vi "Register.vi"(8 "error in (no error)":errorcluster, 11 "Test Executive Builder Model in":refnum<class "Test Executive Builder Model.lvclass">) -> (0 "error out":errorcluster, 3 "Test Executive Builder Model out":refnum<class "Test Executive Builder Model.lvclass">)   [LabVIEW 2017, in "Test Executive Builder Model.lvclass"]
uses:
  Test Executive Builder Model.lvclass
  Test Executive Builder Model Messages/Load Test Executive Msg/Load Test Executive Msg.lvclass
  <vilib>/gpm_packages/@cs/mva-core/Source/IObserver/IObserver/IObserver.lvclass
  <vilib>/gpm_packages/@cs/mva-core/Source/SubscriptionPolicy/BasicSubscription/BasicSubscription.lvclass
  Test Executive Builder Model Messages/Insert While Loop Msg/Insert While Loop Msg.lvclass
  Application Dependencies/Insert While Loop.ctl
  Test Executive Builder Model Messages/Insert For Loop Msg/Insert For Loop Msg.lvclass
  Application Dependencies/Insert For Loop.ctl
  Test Executive Builder Model Messages/Insert Stop Loop Msg/Insert Stop Loop Msg.lvclass
  Application Dependencies/Insert Stop Loop.ctl
  Test Executive Builder Model Messages/Insert Test Step Msg/Insert Test Step Msg.lvclass
  Application Dependencies/Insert Test Step.ctl
  Test Executive Builder Model Messages/Insert Subroutine Msg/Insert Subroutine Msg.lvclass
  Application Dependencies/Insert Subroutine.ctl
  Test Executive Builder Model Messages/Insert Subsequence Msg/Insert Subsequence Msg.lvclass
  Application Dependencies/Insert Subsequence.ctl
  Test Executive Builder Model Messages/Insert Conditional Msg/Insert Conditional Msg.lvclass
  Application Dependencies/Insert Conditional.ctl
  Test Executive Builder Model Messages/Remove Element Msg/Remove Element Msg.lvclass
  Test Executive Builder Model Messages/Move or Copy Element Msg/Move or Copy Element Msg.lvclass
  Application Dependencies/Move or Copy Element.ctl
  Test Executive Builder Model Messages/Save Test Executive Msg/Save Test Executive Msg.lvclass
  Test Executive Builder Model Messages/Clear Test Executive Msg/Clear Test Executive Msg.lvclass
  Test Executive Builder Model Messages/Create Test Executive Msg/Create Test Executive Msg.lvclass
  Application Dependencies/Create Test Executive.ctl
  Test Executive Builder Model Messages/Handle Double Click on Element Msg/Handle Double Click on Element Msg.lvclass
  Test Executive Builder Model Messages/Drop Element Msg/Drop Element Msg.lvclass
  Application Dependencies/Drop Element.ctl
  Application Dependencies/Insert Case Structure.ctl
  Test Executive Builder Model Messages/Insert Case Structure Msg/Insert Case Structure Msg.lvclass
  Application Dependencies/Insert Halt.ctl
  Test Executive Builder Model Messages/Insert Halt Msg/Insert Halt Msg.lvclass
  Test Executive Builder Model Messages/Mass Relink Msg/Mass Relink Msg.lvclass
  Test Executive Builder Model Messages/Insert Parallel Msg/Insert Parallel Msg.lvclass
  C:/Program Files/National Instruments/LabVIEW 2017/vi.lib/gpm_packages/@cs/mva-core/Source/IModel/IModel/IModel.lvclass
  C:/Program Files/National Instruments/LabVIEW 2017/vi.lib/gpm_packages/@cs/mva-core/Source/IObserver/IObserver/IObserver.lvclass
  C:/Program Files/National Instruments/LabVIEW 2017/vi.lib/ActorFramework/Actor/Actor.lvclass
  Application Dependencies/Insert Parallel.ctl
  C:/Program Files/National Instruments/LabVIEW 2017/vi.lib/gpm_packages/@cs/mva-core/Source/IMediator/ISubscriptionPolicy/ISubscriptionPolicy.lvclass
  C:/Program Files/National Instruments/LabVIEW 2017/vi.lib/gpm_packages/@cs/transport/Source/Concrete/ActorMessageTransport/Notification Msg/Notification Msg.lvclass
  C:/Program Files/National Instruments/LabVIEW 2017/vi.lib/gpm_packages/@cs/actor-framework-messages/Source/RoundTripMessage/RoundTripMessage.lvclass
  C:/Program Files/National Instruments/LabVIEW 2017/vi.lib/ActorFramework/Message/Message.lvclass
  <vilib>/gpm_packages/@cs/transport/Source/Concrete/ActorMessageTransport/Notification Msg/Notification Msg.lvclass
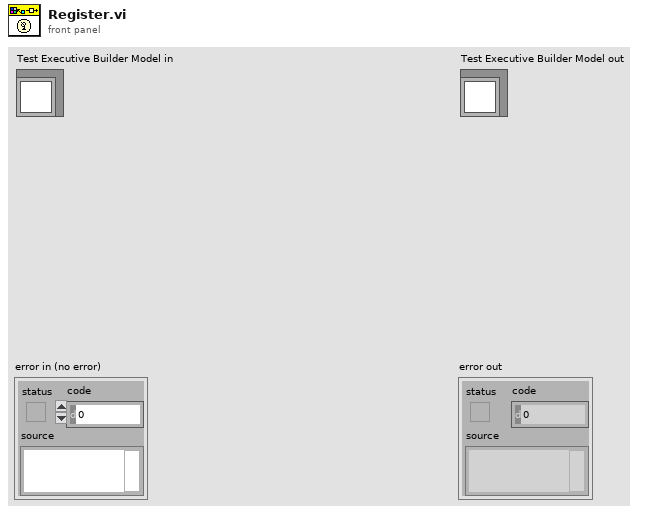
[diagram p1: front panel]
types:
  T1 = typedef "Insert Parallel.ctl" = cluster{"Parent ID":string, "Insertion Index":i32}
  T2 = typedef "Insert Halt.ctl" = cluster{"Parent ID":string, "Insertion Index":i32}
  T3 = typedef "Insert Case Structure.ctl" = cluster{"Parent ID":string, "Insertion Index":i32}
  T4 = typedef "Drop Element.ctl" = cluster{"Parent ID":string, "Insertion Index":i32, "Tag":string, "Ctrl":bool}
  T5 = typedef "Create Test Executive.ctl" = cluster{"Folder Path":path, "File Name with Extension":string}
  T6 = typedef "Move or Copy Element.ctl" = cluster{"Parent ID":string, "Insertion Index":i32, "Tag":string, "Ctrl":bool}
  T7 = typedef "Insert Conditional.ctl" = cluster{"Parent ID":string, "Insertion Index":i32}
  T8 = typedef "Insert Subsequence.ctl" = cluster{"Parent ID":string, "Insertion Index":i32}
  T9 = typedef "Insert Subroutine.ctl" = cluster{"Parent ID":string, "Insertion Index":i32, "Path":path}
  T10 = typedef "Insert Test Step.ctl" = cluster{"Parent ID":string, "Insertion Index":i32, "Test Step":string}
  T11 = typedef "Insert Stop Loop.ctl" = cluster{"Parent ID":string, "Insertion Index":i32}
  T12 = typedef "Insert For Loop.ctl" = cluster{"Parent ID":string, "Insertion Index":i32, "Iterations":i32}
  T13 = typedef "Insert While Loop.ctl" = cluster{"Parent ID":string, "Insertion Index":i32}
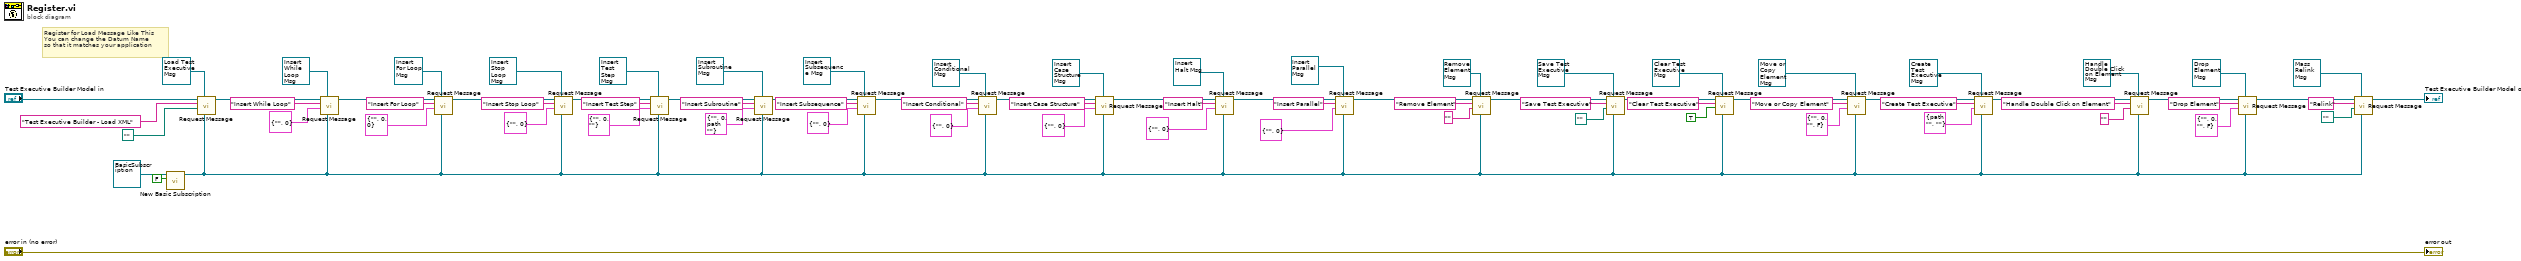
[diagram p0: block diagram]
diagram:
  # "Register for Load Message Like This\nYou can change the Datum Name \nso that it matches your application"
  n1 = call <vilib>:"New Basic Subscription.vi"("Ignore Past Updates? (F)"=FALSE, "BasicSubscription In"=refnum<class "BasicSubscription.lvclass"> refnum ("SubscriptionPolicy.lvlib:BasicSubscription.lvclass")) -> ("BasicSubscription Out"=w2:refnum<class "BasicSubscription.lvclass">)  [unwired: 9 in]
  n2 = call <vilib>:"Request Message.vi"("Configured SubscriptionPolicy"=w2, "Desired Notification Msg"=refnum<class "Load Test Executive Msg.lvclass"> refnum ("Test Executive Builder Model.lvlib:Load Test Executive Msg.lvclass"), "Data Type"=path "", "Datum Name"="Test Executive Builder - Load XML", "IObserver in"="Test Executive Builder Model in") -> ("IObserver out"=w71:refnum<class "Test Executive Builder Model.lvclass">)  [unwired: 4 in, 2 out]
  n3 = call <vilib>:"Request Message.vi"("Configured SubscriptionPolicy"=w2, "Desired Notification Msg"=refnum<class "Insert While Loop Msg.lvclass"> refnum ("Test Executive Builder Model.lvlib:Insert While Loop Msg.lvclass"), "Data Type"=T13 {"Parent ID"="", "Insertion Index"=0} ("Insert While Loop"), "Datum Name"="Insert While Loop", "IObserver in"=w71) -> ("IObserver out"=w69:refnum<class "Test Executive Builder Model.lvclass">)  [unwired: 4 in, 2 out]
  n4 = call <vilib>:"Request Message.vi"("Configured SubscriptionPolicy"=w2, "Desired Notification Msg"=refnum<class "Insert For Loop Msg.lvclass"> refnum ("Test Executive Builder Model.lvlib:Insert For Loop Msg.lvclass"), "Data Type"=T12 {"Parent ID"="", "Insertion Index"=0, "Iterations"=0} ("Insert For Loop"), "Datum Name"="Insert For Loop", "IObserver in"=w69) -> ("IObserver out"=w65:refnum<class "Test Executive Builder Model.lvclass">)  [unwired: 4 in, 2 out]
  n5 = call <vilib>:"Request Message.vi"("Configured SubscriptionPolicy"=w2, "Desired Notification Msg"=refnum<class "Insert Stop Loop Msg.lvclass"> refnum ("Test Executive Builder Model.lvlib:Insert Stop Loop Msg.lvclass"), "Data Type"=T11 {"Parent ID"="", "Insertion Index"=0} ("Insert Stop Loop"), "Datum Name"="Insert Stop Loop", "IObserver in"=w65) -> ("IObserver out"=w61:refnum<class "Test Executive Builder Model.lvclass">)  [unwired: 4 in, 2 out]
  n6 = call <vilib>:"Request Message.vi"("Configured SubscriptionPolicy"=w2, "Desired Notification Msg"=refnum<class "Insert Test Step Msg.lvclass"> refnum ("Test Executive Builder Model.lvlib:Insert Test Step Msg.lvclass"), "Data Type"=T10 {"Parent ID"="", "Insertion Index"=0, "Test Step"=""} ("Insert Test Step"), "Datum Name"="Insert Test Step", "IObserver in"=w61) -> ("IObserver out"=w57:refnum<class "Test Executive Builder Model.lvclass">)  [unwired: 4 in, 2 out]
  n7 = call <vilib>:"Request Message.vi"("Configured SubscriptionPolicy"=w2, "Desired Notification Msg"=refnum<class "Insert Subroutine Msg.lvclass"> refnum ("Test Executive Builder Model.lvlib:Insert Subroutine Msg.lvclass"), "Data Type"=T9 {"Parent ID"="", "Insertion Index"=0, "Path"=path ""} ("Insert Subroutine"), "Datum Name"="Insert Subroutine", "IObserver in"=w57) -> ("IObserver out"=w53:refnum<class "Test Executive Builder Model.lvclass">)  [unwired: 4 in, 2 out]
  n8 = call <vilib>:"Request Message.vi"("Configured SubscriptionPolicy"=w2, "Desired Notification Msg"=refnum<class "Insert Subsequence Msg.lvclass"> refnum ("Test Executive Builder Model.lvlib:Insert Subsequence Msg.lvclass"), "Data Type"=T8 {"Parent ID"="", "Insertion Index"=0} ("Insert Subsequence"), "Datum Name"="Insert Subsequence", "IObserver in"=w53) -> ("IObserver out"=w49:refnum<class "Test Executive Builder Model.lvclass">)  [unwired: 4 in, 2 out]
  n9 = call <vilib>:"Request Message.vi"("Configured SubscriptionPolicy"=w2, "Desired Notification Msg"=refnum<class "Insert Conditional Msg.lvclass"> refnum ("Test Executive Builder Model.lvlib:Insert Conditional Msg.lvclass"), "Data Type"=T7 {"Parent ID"="", "Insertion Index"=0} ("Insert Conditional"), "Datum Name"="Insert Conditional", "IObserver in"=w49) -> ("IObserver out"=w17:refnum<class "Test Executive Builder Model.lvclass">)  [unwired: 4 in, 2 out]
  n10 = call <vilib>:"Request Message.vi"("Configured SubscriptionPolicy"=w2, "Desired Notification Msg"=refnum<class "Insert Case Structure Msg.lvclass"> refnum ("Insert Case Structure Msg.lvclass"), "Data Type"=T3 {"Parent ID"="", "Insertion Index"=0} ("Insert Case Structure"), "Datum Name"="Insert Case Structure", "IObserver in"=w17) -> ("IObserver out"=w14:refnum<class "Test Executive Builder Model.lvclass">)  [unwired: 4 in, 2 out]
  n11 = call <vilib>:"Request Message.vi"("Configured SubscriptionPolicy"=w2, "Desired Notification Msg"=refnum<class "Insert Halt Msg.lvclass"> refnum ("Insert Halt Msg.lvclass"), "Data Type"=T2 {"Parent ID"="", "Insertion Index"=0} ("Insert Halt"), "Datum Name"="Insert Halt", "IObserver in"=w14) -> ("IObserver out"=w4:refnum<class "Test Executive Builder Model.lvclass">)  [unwired: 4 in, 2 out]
  n12 = call <vilib>:"Request Message.vi"("Configured SubscriptionPolicy"=w2, "Desired Notification Msg"=refnum<class "Insert Parallel Msg.lvclass"> refnum ("Insert Parallel Msg.lvclass"), "Data Type"=T1 {"Parent ID"="", "Insertion Index"=0} ("Insert Parallel"), "Datum Name"="Insert Parallel", "IObserver in"=w4) -> ("IObserver out"=w3:refnum<class "Test Executive Builder Model.lvclass">)  [unwired: 4 in, 2 out]
  n13 = call <vilib>:"Request Message.vi"("Configured SubscriptionPolicy"=w2, "Desired Notification Msg"=refnum<class "Remove Element Msg.lvclass"> refnum ("Test Executive Builder Model.lvlib:Remove Element Msg.lvclass"), "Data Type"="", "Datum Name"="Remove Element", "IObserver in"=w3) -> ("IObserver out"=w38:refnum<class "Test Executive Builder Model.lvclass">)  [unwired: 4 in, 2 out]
  n14 = call <vilib>:"Request Message.vi"("Configured SubscriptionPolicy"=w2, "Desired Notification Msg"=refnum<class "Save Test Executive Msg.lvclass"> refnum ("Test Executive Builder Model.lvlib:Save Test Executive Msg.lvclass"), "Data Type"=path "", "Datum Name"="Save Test Executive", "IObserver in"=w38) -> ("IObserver out"=w40:refnum<class "Test Executive Builder Model.lvclass">)  [unwired: 4 in, 2 out]
  n15 = call <vilib>:"Request Message.vi"("Configured SubscriptionPolicy"=w2, "Desired Notification Msg"=refnum<class "Clear Test Executive Msg.lvclass"> refnum ("Test Executive Builder Model.lvlib:Clear Test Executive Msg.lvclass"), "Data Type"=TRUE, "Datum Name"="Clear Test Executive", "IObserver in"=w40) -> ("IObserver out"=w39:refnum<class "Test Executive Builder Model.lvclass">)  [unwired: 4 in, 2 out]
  n16 = call <vilib>:"Request Message.vi"("Configured SubscriptionPolicy"=w2, "Desired Notification Msg"=refnum<class "Move or Copy Element Msg.lvclass"> refnum ("Test Executive Builder Model.lvlib:Move or Copy Element Msg.lvclass"), "Data Type"=T6 {"Parent ID"="", "Insertion Index"=0, "Tag"="", "Ctrl"=FALSE} ("Move or Copy Element"), "Datum Name"="Move or Copy Element", "IObserver in"=w39) -> ("IObserver out"=w29:refnum<class "Test Executive Builder Model.lvclass">)  [unwired: 4 in, 2 out]
  n17 = call <vilib>:"Request Message.vi"("Configured SubscriptionPolicy"=w2, "Desired Notification Msg"=refnum<class "Create Test Executive Msg.lvclass"> refnum ("Test Executive Builder Model.lvlib:Create Test Executive Msg.lvclass"), "Data Type"=T5 {"Folder Path"=path "", "File Name with Extension"=""} ("Create Test Executive"), "Datum Name"="Create Test Executive", "IObserver in"=w29) -> ("IObserver out"=w26:refnum<class "Test Executive Builder Model.lvclass">)  [unwired: 4 in, 2 out]
  n18 = call <vilib>:"Request Message.vi"("Configured SubscriptionPolicy"=w2, "Desired Notification Msg"=refnum<class "Handle Double Click on Element Msg.lvclass"> refnum ("Test Executive Builder Model.lvlib:Handle Double Click on Element Msg.lvclass"), "Data Type"="", "Datum Name"="Handle Double Click on Element", "IObserver in"=w26) -> ("IObserver out"=w22:refnum<class "Test Executive Builder Model.lvclass">)  [unwired: 4 in, 2 out]
  n19 = call <vilib>:"Request Message.vi"("Configured SubscriptionPolicy"=w2, "Desired Notification Msg"=refnum<class "Drop Element Msg.lvclass"> refnum ("Test Executive Builder Model.lvlib:Drop Element Msg.lvclass"), "Data Type"=T4 {"Parent ID"="", "Insertion Index"=0, "Tag"="", "Ctrl"=FALSE} ("Drop Element"), "Datum Name"="Drop Element", "IObserver in"=w22) -> ("IObserver out"=w10:refnum<class "Test Executive Builder Model.lvclass">)  [unwired: 4 in, 2 out]
  n20 = call <vilib>:"Request Message.vi"("Configured SubscriptionPolicy"=w2, "Desired Notification Msg"=refnum<class "Mass Relink Msg.lvclass"> refnum ("Mass Relink Msg.lvclass"), "Data Type"=path "", "Datum Name"="Relink", "IObserver in"=w10) -> ("IObserver out"=→"Test Executive Builder Model out":refnum<class "Test Executive Builder Model.lvclass">)  [unwired: 4 in, 2 out]
  "error out" <- "error in (no error)"
